vi "PM100D Measure1.vi"() -> (4 "Read Power#1":string, 6 "Read Power#2":string, 8 "Readout value#1":dbl format="%^#_6e", 10 "Readout value#2":dbl format="%^#_6e")   [LabVIEW 2020]
doc: "This VI shows how to communicate with a PM100D optical power/energy meter with SCPI commands.\n- Initializing the instrument\n- Getting system info\n- Setting parameters\n- Measurement configuration\n- Measuring queue\n- Fetching and displaying a measurement value\n- Closing the application"
panel:
  in  "Enum":enum16{"0", "1", "2", "3", "4"}(ring)
  out "Error log 2":string
  out "Sensor Name 2":string
  out "Sensor SN 2":string
  out "Power Meter#2":string
  out "Power Meter#1":string
  out "Sensor SN":string
  out "Sensor Name":string
  out "New":bool
  in  "Timeout [ms]":i32=1000
  in  "stop":bool
  in  "Readout Config":string(combo)="POW"
  out "Error log":string
  in  "Averaging Rate":i32=300
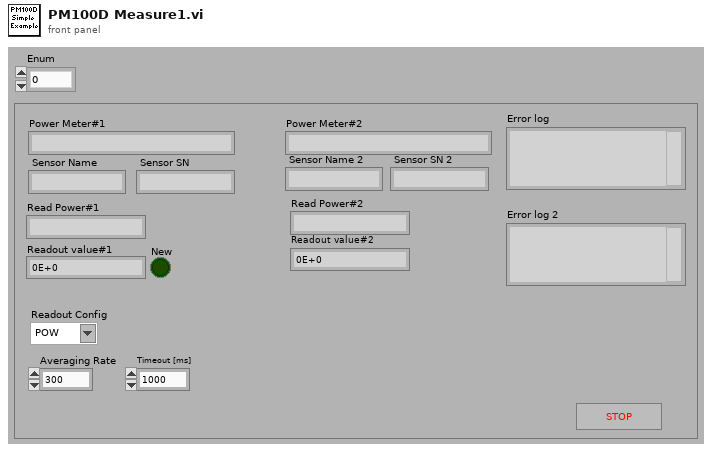
[diagram p1: front panel]
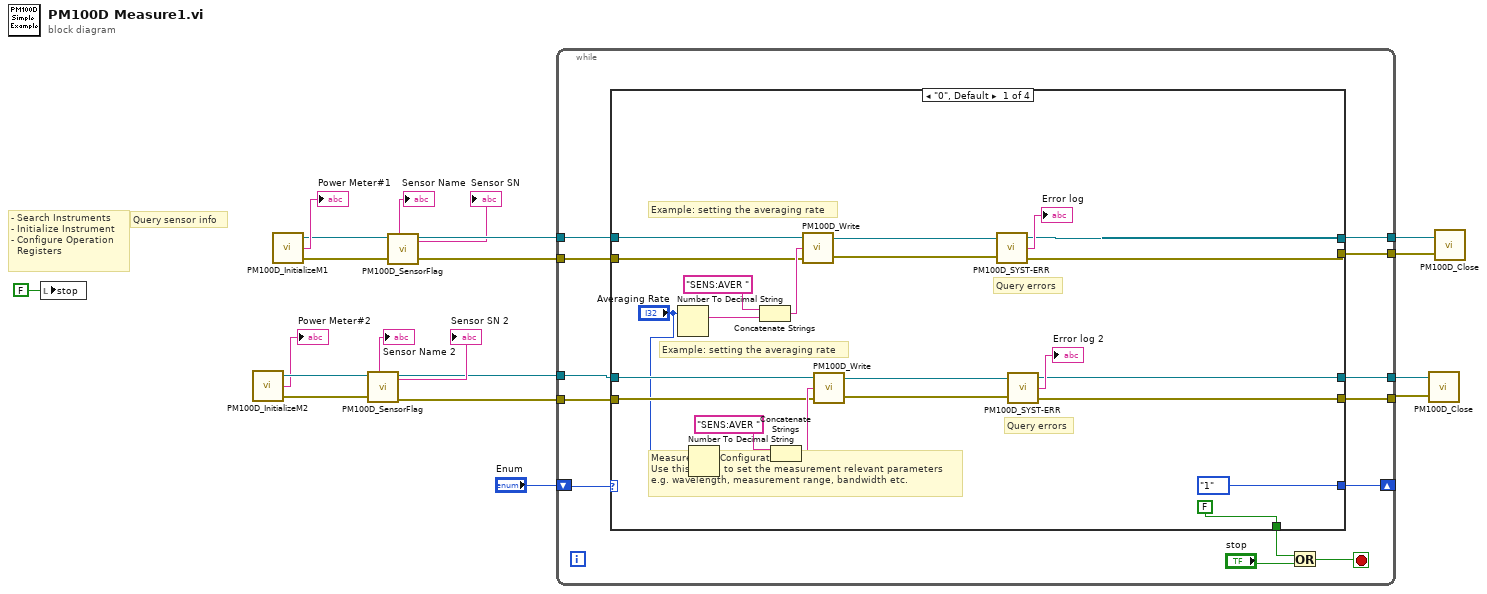
[diagram p0: block diagram]
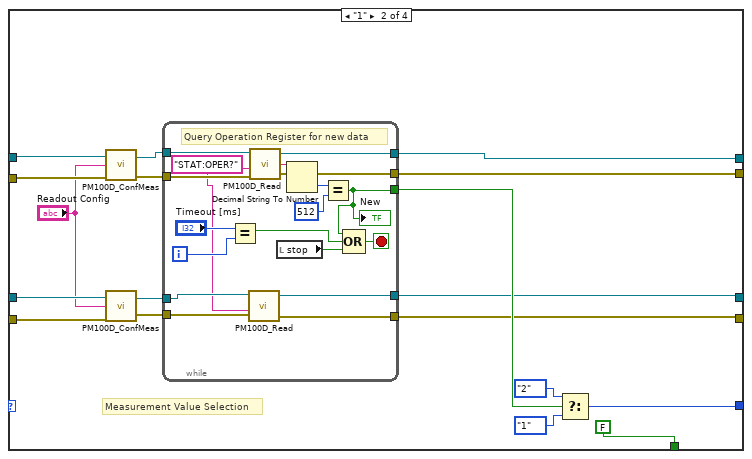
[diagram p2: hidden frame]
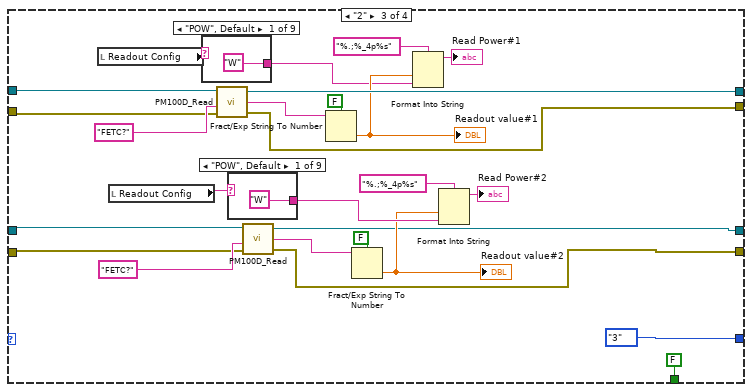
[diagram p3: hidden frame]
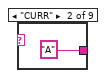
[diagram p4: hidden frame]
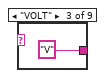
[diagram p5: hidden frame]
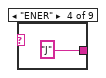
[diagram p6: hidden frame]
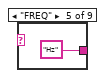
[diagram p7: hidden frame]
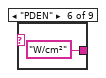
[diagram p8: hidden frame]
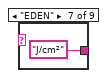
[diagram p9: hidden frame]
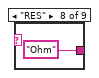
[diagram p10: hidden frame]
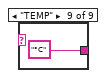
[diagram p11: hidden frame]
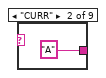
[diagram p12: hidden frame]
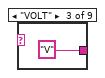
[diagram p13: hidden frame]
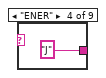
[diagram p14: hidden frame]
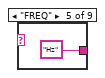
[diagram p15: hidden frame]
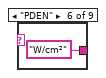
[diagram p16: hidden frame]
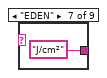
[diagram p17: hidden frame]
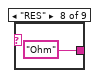
[diagram p18: hidden frame]
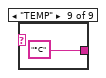
[diagram p19: hidden frame]
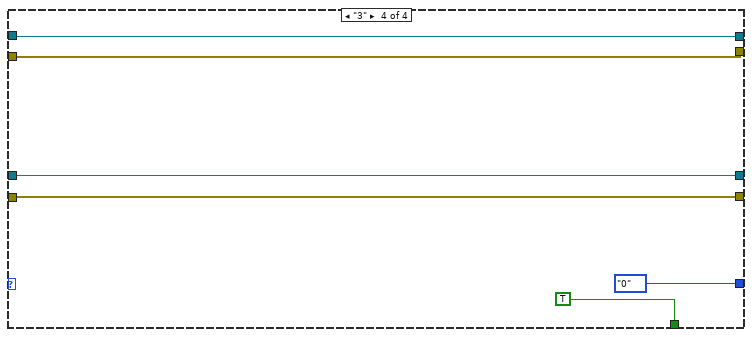
[diagram p20: hidden frame]
diagram:
  # "- Search Instruments\n- Initialize Instrument\n- Configure Operation\n  Registers"
  # "Query sensor info"
  n1 = local write "stop"(FALSE ("stop")) -> ()
  n2 = call "PM100D_InitializeM2.vi"() -> ("error out"=w5:errorcluster, "Instrument"=→"Power Meter#2":string, "VISA out"=w9:refnum<visa-resource-name>)  [unwired: 2 in, 1 out]
  n3 = call "PM100D_InitializeM1.vi"() -> ("error out"=w20:errorcluster, "Instrument"=→"Power Meter#1":string, "VISA out"=w10:refnum<visa-resource-name>)  [unwired: 2 in, 1 out]
  n4 = call "PM100D_SensorFlag.vi"("error in (no error)"=w5, "VISA in"=w9) -> ("error out"=w3:errorcluster, "VISA out"=w4:refnum<visa-resource-name>, "sn"=→"Sensor SN 2":string, "name"=→"Sensor Name 2":string)  [unwired: 2 in, 4 out]
  n5 = call "PM100D_SensorFlag.vi"("error in (no error)"=w20, "VISA in"=w10) -> ("error out"=w18:errorcluster, "VISA out"=w19:refnum<visa-resource-name>, "sn"=→"Sensor SN":string, "name"=→"Sensor Name":string)  [unwired: 2 in, 4 out]
  n6 = while {
    tunnel: w19 -> [w33]
    tunnel: w18 -> [w32]
    shift-right: [w30] -> _
    shift-left: "Enum" -> [w31]
    tunnel: [w29] -> w13
    tunnel: [w28] -> w12
    tunnel: w4 -> [w27]
    tunnel: w3 -> [w26]
    tunnel: [w25] -> w2
    tunnel: [w24] -> w1
    stop <- w23 stop-if-true
    n7 = case shown="\"0\", Default" w31 {
      tunnel: w33 -> [w54 w74 w117 w142]
      tunnel: w32 -> [w49 w73 w116 w141]
      tunnel: [enum16{"0", "1", "2"}."1" w68 enum16{"0", "1", "2", "3", "4"}."3" enum16{"0", "1", "2", "3", "4"}."0" ("f")] -> w30
      tunnel: [w47 w70 w115 w142] -> w29
      tunnel: [w46 w69 w107 w141] -> w28
      tunnel: w27 -> [w39 w64 w98 w140]
      tunnel: w26 -> [w38 w62 w97 w139]
      tunnel: [w37 w59 w95 w140] -> w25
      tunnel: [w36 w58 w96 w139] -> w24
      tunnel: [FALSE ("stop") FALSE ("stop") FALSE ("stop") TRUE ("stop")] -> w21
      frame "0", Default {
        # "Query errors"
        # "Example: setting the averaging rate"
        # "Query errors"
        # "Example: setting the averaging rate"
        # "Measurement Configuration\nUse this frame to set the measurement relevant parameters\ne.g. wavelength, measurement range, bandwidth etc."
        n8 = Number To Decimal String(number="Averaging Rate") -> (decimal integer string=w55:string)  [unwired: 1 in]
        n9 = Number To Decimal String(number="Averaging Rate") -> (decimal integer string=w41:string)  [unwired: 1 in]
        n10 = Concatenate Strings("SENS:AVER " ("string"), w55) -> (w53:string)
        n11 = Concatenate Strings("SENS:AVER " ("string"), w41) -> (w42:string)
        n12 = call "PM100D_Write.vi"("error in (no error)"=w49, "Command"=w53, "VISA in"=w54) -> ("error out"=w50:errorcluster, "VISA out"=w52:refnum<visa-resource-name>)
        n13 = call "PM100D_Write.vi"("error in (no error)"=w38, "Command"=w42, "VISA in"=w39) -> ("error out"=w45:errorcluster, "VISA out"=w43:refnum<visa-resource-name>)
        n14 = call "PM100D_SYST-ERR.vi"("error out 2"=w50, "VISA In"=w52) -> ("error out"=w46:errorcluster, "Error"=→"Error log":string, "VISA Out"=w47:refnum<visa-resource-name>)  [unwired: 1 in]
        n15 = call "PM100D_SYST-ERR.vi"("error out 2"=w45, "VISA In"=w43) -> ("error out"=w36:errorcluster, "Error"=→"Error log 2":string, "VISA Out"=w37:refnum<visa-resource-name>)  [unwired: 1 in]
      }
      frame "1" {
        # "Measurement Value Selection"
        n16 = call "PM100D_ConfMeas.vi"("error in"=w73, "Conf:"="Readout Config", "VISA In"=w74) -> ("error out"=w71:errorcluster, "dup VISA session"=w72:refnum<visa-resource-name>)
        n17 = call "PM100D_ConfMeas.vi"("error in"=w62, "Conf:"="Readout Config", "VISA In"=w64) -> ("error out"=w60:errorcluster, "dup VISA session"=w61:refnum<visa-resource-name>)
        n18 = while {
          tunnel: w72 -> [w89]
          tunnel: w71 -> [w88]
          tunnel: [w87] -> w70
          tunnel: [w86] -> w69
          tunnel: [w80] -> w65
          tunnel: w61 -> [w79]
          tunnel: w60 -> [w78]
          tunnel: [w76] -> w59
          tunnel: [w75] -> w58
          i -> [w82]
          stop <- w84 stop-if-true
          w77 = "STAT:OPER?" ("Command")
          # "Query Operation Register for new data"
          n19 = Equal?(x="Timeout [ms]", y=w82) -> (x = y?=w81:bool)
          n20 = call "PM100D_Read.vi"("error in (no error)"=w78, "Command"=w77, "VISA in"=w79) -> ("error out"=w75:errorcluster, "VISA out"=w76:refnum<visa-resource-name>)  [unwired: 1 in, 1 out]
          n21 = call "PM100D_Read.vi"("error in (no error)"=w88, "Command"=w77, "VISA in"=w89) -> ("error out"=w86:errorcluster, "ReadValue"=w92:string, "VISA out"=w87:refnum<visa-resource-name>)  [unwired: 1 in]
          n22 = local read "stop"() -> (w85:bool)
          n23 = Decimal String To Number(string=w92) -> (number=w91:i32)  [unwired: 2 in, 1 out]
          n24 = Equal?(x=w91, y=512) -> (x = y?=w80:bool)
          "New" <- w80
          n25 = Compound Arithmetic op=OR(w80, w81, w85) -> (w84:bool)
        }
        n26 = Select(t=enum16{"0", "1", "2"}."2", s=w65, f=enum16{"0", "1", "2"}."1") -> (s? t:f=w68:enum16{"0", "1", "2"})
      }
      frame "2" {
        n27 = local read "Readout Config"() -> (w114:string)
        n28 = local read "Readout Config"() -> (w100:string)
        n29 = case shown="\"POW\", Default" w114 {
          tunnel: ["W" "A" "V" "J" "Hz" "W/cm²" "J/cm²" "Ohm" "°C"] -> w109
          frame "POW", Default {
          }
          frame "CURR" {
          }
          frame "VOLT" {
          }
          frame "ENER" {
          }
          frame "FREQ" {
          }
          frame "PDEN" {
          }
          frame "EDEN" {
          }
          frame "RES" {
          }
          frame "TEMP" {
          }
        }
        n30 = call "PM100D_Read.vi"("error in (no error)"=w116, "Command"="FETC?", "VISA in"=w117) -> ("error out"=w107:errorcluster, "ReadValue"=w113:string, "VISA out"=w115:refnum<visa-resource-name>)  [unwired: 1 in]
        n31 = case shown="\"POW\", Default" w100 {
          tunnel: ["W" "A" "V" "J" "Hz" "W/cm²" "J/cm²" "Ohm" "°C"] -> w105
          frame "POW", Default {
          }
          frame "CURR" {
          }
          frame "VOLT" {
          }
          frame "ENER" {
          }
          frame "FREQ" {
          }
          frame "PDEN" {
          }
          frame "EDEN" {
          }
          frame "RES" {
          }
          frame "TEMP" {
          }
        }
        n32 = call "PM100D_Read.vi"("error in (no error)"=w97, "Command"="FETC?", "VISA in"=w98) -> ("error out"=w96:errorcluster, "ReadValue"=w101:string, "VISA out"=w95:refnum<visa-resource-name>)  [unwired: 1 in]
        n33 = Fract/Exp String To Number(use system decimal point (T)=FALSE, string=w113) -> (number=w110:dbl)  [unwired: 2 in, 1 out]
        "Readout value#1" <- w110
        n34 = Fract/Exp String To Number(use system decimal point (T)=FALSE, string=w101) -> (number=w104:dbl)  [unwired: 2 in, 1 out]
        "Readout value#2" <- w104
        n35 = Format Into String(format string="%.;%_4p%s", w110, w109) -> (resulting string=→"Read Power#1":string)  [unwired: 2 in, 1 out]
        n36 = Format Into String(format string="%.;%_4p%s", w104, w105) -> (resulting string=→"Read Power#2":string)  [unwired: 2 in, 1 out]
      }
      frame "3" {
      }
    }
    n37 = Or(x=w21, y="stop") -> (x .or. y?=w23:bool)
  }
  n38 = call "PM100D_Close.vi"("error in (no error)"=w1, "VISA resource name"=w2) -> ()  [unwired: 2 in]
  n39 = call "PM100D_Close.vi"("error in (no error)"=w12, "VISA resource name"=w13) -> ()  [unwired: 2 in]
